vi "SpecFilter.vi"() -> ()   [LabVIEW 2022 SP3]
uses:
  <vilib>/Analysis/NI_AALPro.lvlib
  <vilib>/Analysis/NI_AALBase.lvlib
  <vilib>/Analysis/2dsp.llb/Real FFT.vi
  <vilib>/Analysis/baseanly.llb/Mean (DBL).vi
panel:
  out "Stats":T1 {"Raw ratio" format="%.2f"; "Spec Ratio" format="%.2f"; "Spec SD" format="%.2f"; "Spec mean" format="%.2f"; "Raw SD" format="%.2f"; "Raw mean" format="%.2f"}
  out "Raw Envelope":dbl[][](array[numeric]) format="%.2f"
  out "Spec Data":dbl[][](array[numeric]) format="%.2f"
  out "XY Graph":T2(graph)
  out "Specle Sector image":dbl[][](graph)
  out "Specle Image":dbl[][](graph)
  in  "Log scaling?":bool=TRUE
  in  "Last file opened":path
  out "Sector as data array":dbl[][](graph)
  in  "View Header?":bool
  in  "Header format":u16(ring) items=["Riverside Format", "Ron Linear"]
  out "Raw data":i16[][](graph)
  in  "new file path":path=path "E:/ProstateData/Q162r19.eye"
  # "To view new EYE file delete file path, run application by pushing right pointing arrow, and then choose new file in dialog box."
  # "Ignore if not using a sector scan"
  # "Note columns of the raw data have been inverted\nand the resulting matrix has been transposed to form\nthe sector image. Data reduced from raw form"
  # "© 2000 Riverside Research Institute"
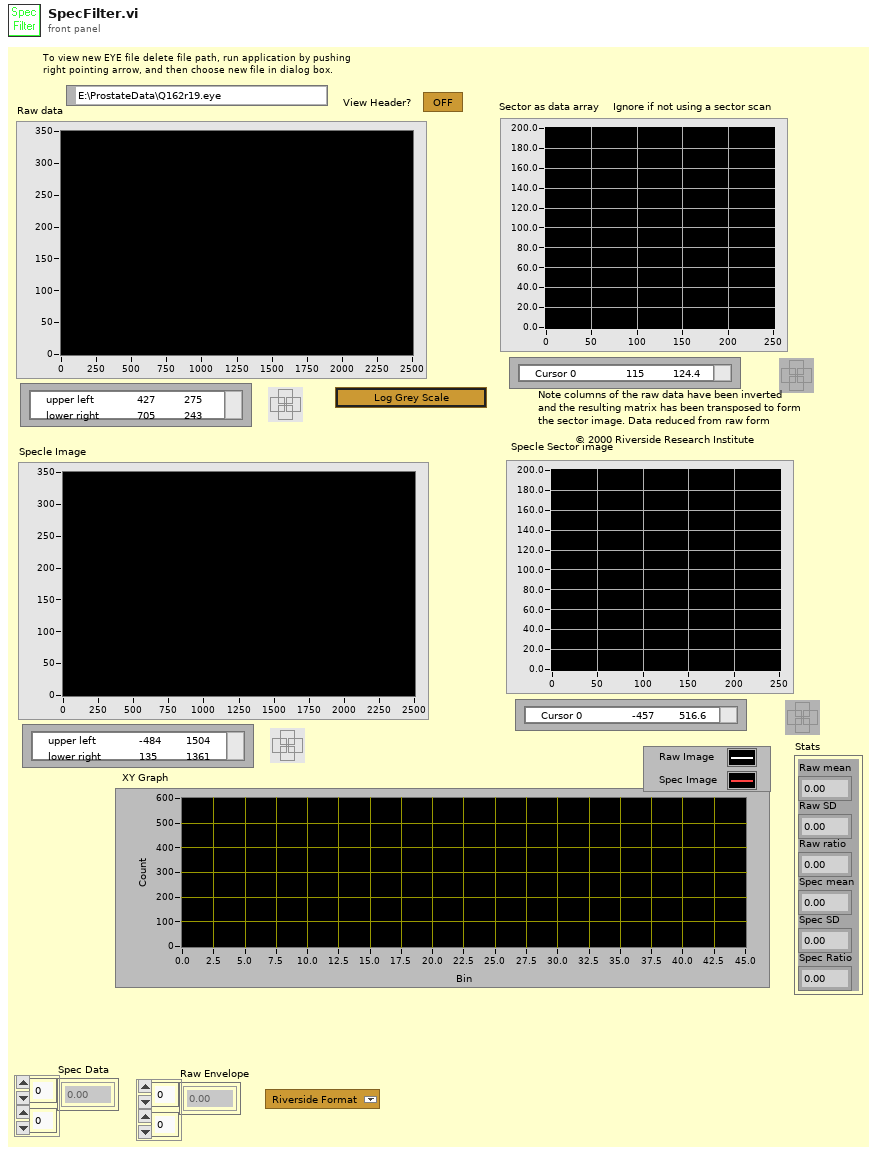
[diagram p1: front panel]
types:
  T1 = cluster{"Raw mean":dbl, "Raw SD":dbl, "Raw ratio":dbl, "Spec mean":dbl, "Spec SD":dbl, "Spec Ratio":dbl}
  T2 = cluster{"X Values":dbl[], "Histogram: h(x)":i32[]}[]
  T3 = cluster{"# rf points per line":u16, "# lines per scan":u16, "sample rate MHz":u16, "# A/D bits":u16, "# bytes per A/D":u16, "TGC Flag":u16, "A/D Type":string}
  T4 = cluster{"bandwidth":sgl, "center freq":sgl, "start freq":sgl, "ID":i32}
  T5 = cluster{"delay":sgl, "pivot distance":sgl, "sector scan angle":sgl, "operator":string, "Scan Mode":string, "location":string}
  T6 = cluster{"X Values":dbl[], "Histogram: h(x)":i32[]}
  T7 = cluster{"mean":dbl, "standard deviation":dbl, dbl, "mean":dbl, "standard deviation":dbl, dbl}
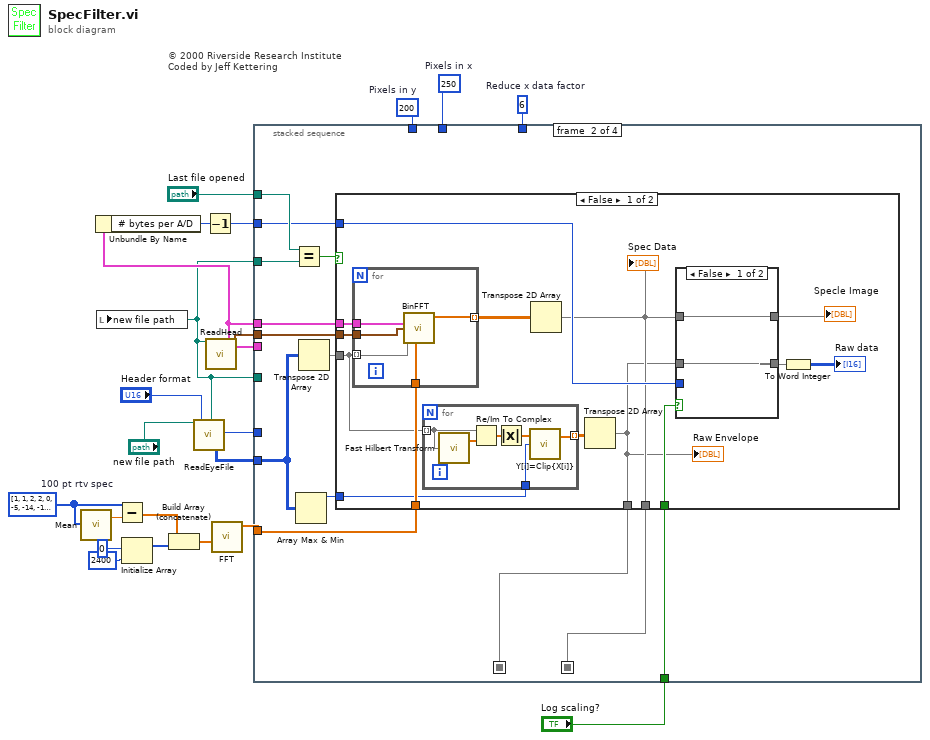
[diagram p0: block diagram]
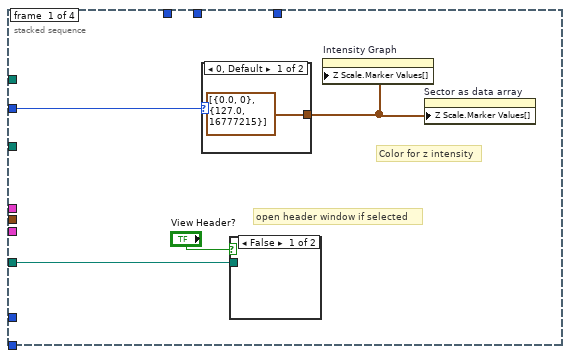
[diagram p2: hidden frame]
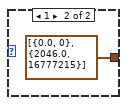
[diagram p3: hidden frame]
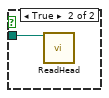
[diagram p4: hidden frame]
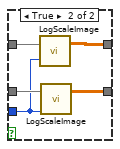
[diagram p5: hidden frame]
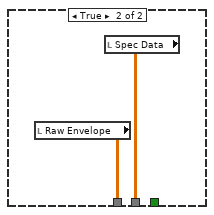
[diagram p6: hidden frame]
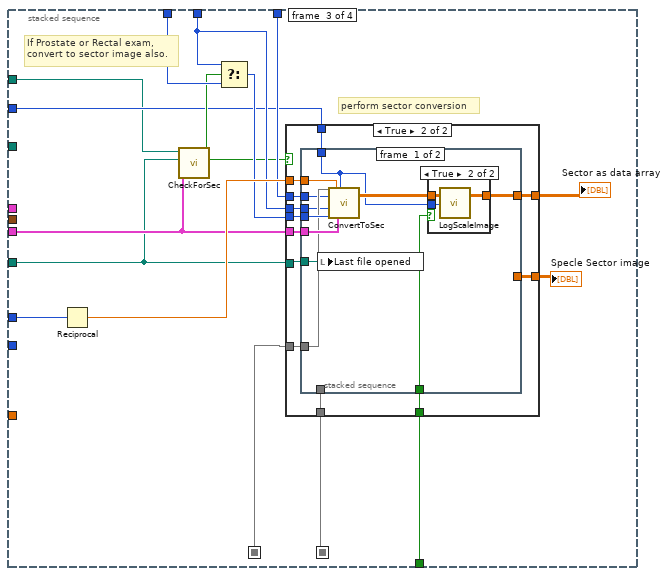
[diagram p7: hidden frame]
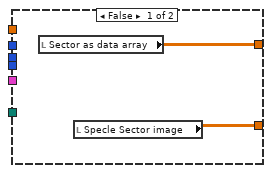
[diagram p8: hidden frame]
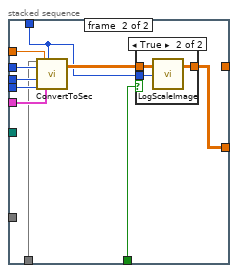
[diagram p10: hidden frame]
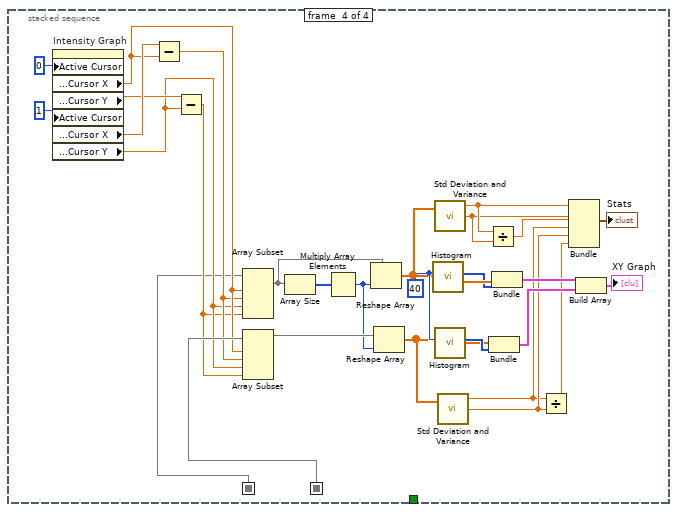
[diagram p12: hidden frame]
diagram:
  w10 = i16[] [1, 1, 2, 2, 0, -5, -14, -15, 1, 31, 52, 42, -4, -58, -81, -58, 2, 62, 88, 70, 20, -31, -56, -51, -27, 3, 20, 22, 14, 6, 0, -3, -5, -6, -7, -6, -3, -2, 0, 2, 3, 2, 1, -1, -3, -4, -3, -2, 1, 2, 2, 2, 1, 0, -1, -1, -1, 0, 1, 1, 1, 1, 1, 1, 1, 0, 0, 0, 0, 0, 1, 1, 1, 1, 1, 0, 0, 0, 0, 1, 1, 1, 1, 1, 1, 1, 1, 0, 0, 1, 1, 1, 1, 1, 1, 0, 0, 0, 0, 0]  # 100 pt rtv spec
  w17 = 6  # Reduce x data factor
  w19 = i16 200  # Pixels in y
  w18 = i16 250  # Pixels in x
  # "© 2000 Riverside Research Institute\nCoded by Jeff Kettering"
  n1 = call-poly <vilib>:"Mean.vi"("X"=w10) -> ("mean"=w12:dbl)  [unwired: 1 out]
  n2 = Subtract(x=w10, y=w12) -> (x-y=w8:dbl[])
  n3 = Initialize Array(0, 2400) -> (w11:i32[])
  n4 = Build Array (concatenate)(w8, w11) -> (w9:dbl[])
  n5 = call "ReadEyeFile.vi"("new file path"="new file path", "Header format"="Header format") -> ("new path out"=w1:path, "2-D data array"=w21:i16[][], "sample rate MHz"=w22:u16)  [unwired: 15 out]
  n6 = local write "new file path"(w1) -> ()
  n7 = call "ReadHead.vi"("new file path"=w1) -> ("A/D info"=w5:T3, "Tranducer Info"=w13:T4, "Scan Info"=w23:T5)  [unwired: 16 out]
  n8 = Unbundle By Name(w5) -> ("# bytes per A/D"=w4:u16)
  n9 = Decrement(x=w4) -> (x-1=w3:u16)
  n10 = call-poly <vilib>:"FFT.vi"("X"=w9) -> ("FFT {X}"=w7:cdb[])  [unwired: 2 in, 8 out]
  n11 = stacked-sequence {
    seq-local: [_ w38 _ _] -> [_ _ w80 w164]
    seq-local: [_ w34 _ _] -> [_ _ w78 w148]
    tunnel: w23 -> [_ _ w88 _]
    tunnel: w22 -> [_ _ w93 _]
    tunnel: w21 -> [_ w32 _ _]
    tunnel: w1 -> [w26 _ w86 _]
    tunnel: w19 -> [_ _ w91 _]
    tunnel: w18 -> [_ _ w90 _]
    tunnel: w17 -> [_ _ w89 _]
    tunnel: w5 -> [_ w43 _ _]
    tunnel: w13 -> [_ w42 _ _]
    tunnel: w7 -> [_ w41 _ _]
    tunnel: "Log scaling?" -> [_ w39 w83 _]
    tunnel: w3 -> [w24 w33 w82 _]
    tunnel: "Last file opened" -> [_ w36 w79 _]
    tunnel: w1 -> [_ w35 _ _]
    frame #0 {
      # "Color for z intensity"
      # "open header window if selected"
      n12 = case shown="0, Default" w24 {
        tunnel: [cluster{dbl, u32}[] [{0.0, 0}, {127.0, 16777215}] ("color scheme 3") cluster{dbl, u32}[] [{0.0, 0}, {2046.0, 16777215}] ("color scheme 3")] -> w25
        frame 0, Default {
        }
        frame 1 {
        }
      }
      n13 = case shown="False" "View Header?" {
        tunnel: w26 -> [_ w30]
        frame False {
        }
        frame True {
          n14 = call "ReadHead.vi"("new file path"=w30) -> ()  [unwired: 19 out]
        }
      }
      n15 = property on="Intensity Graph" class="IntGraph (strict)"("Z Scale.Marker Values[]"=w25) -> ()  [unwired: 2 in, 2 out]
      n16 = property on="Sector as data array" class="IntGraph (strict)"("Z Scale.Marker Values[]"=w25) -> ()  [unwired: 2 in, 2 out]
    }
    frame #1 {
      n17 = Equal?(x=w36, y=w35) -> (x = y?=w37:bool)
      n18 = Array Max & Min(array=w32) -> (max value=w31:i16)  [unwired: 3 out]
      n19 = Transpose 2D Array(2D array=w32) -> (transposed array=w40:i16[][])
      n20 = case shown="False" w37 {
        tunnel: w43 -> [w57 _]
        tunnel: w42 -> [w56 _]
        tunnel: w41 -> [w55 _]
        tunnel: w40 -> [w46 _]
        tunnel: w33 -> [w51 _]
        tunnel: w39 -> [w50 _]
        tunnel: [w48 w77] -> w38
        tunnel: [w47 w76] -> w34
        tunnel: w31 -> [w44 _]
        frame False {
          n21 = for {
            tunnel: w57 -> [w75]
            tunnel: w56 -> [w74]
            tunnel: w55 -> [w73]
            tunnel: w46 -> [w72] mode=indexing
            tunnel: [w71] -> w54 mode=indexing
            n22 = call "BinFFT.vi"("Cal Spectrum"=w73, "RF Data Line"=w72, "Tranducer Info"=w74, "A/D info"=w75) -> ("Envelope of\nOutput bins"=w71:dbl[])  [unwired: 1 in, 6 out]
          }
          n23 = for {
            tunnel: w46 -> [w61] mode=indexing
            tunnel: [w59] -> w45 mode=indexing
            tunnel: w44 -> [w58]
            n24 = call <vilib>:"Fast Hilbert Transform.vi"("X"=w61) -> ("Hilbert{X}"=w62:dbl[])  [unwired: 1 out]
            n25 = Re/Im To Complex(1:w62, 2:w61) -> (0:w63:cdb[])
            n26 = Absolute Value(x=w63) -> (abs(x)=w60:dbl[])
            n27 = call <vilib>:"Y[i]=Clip{X[i]}.vi"("upper limit"=w58, "Input Array"=w60) -> ("Clipped Array"=w59:dbl[])  [unwired: 1 in, 1 out]
          }
          n28 = Transpose 2D Array(2D array=w54) -> (transposed array=w48:dbl[][])
          "Spec Data" <- w48
          n29 = Transpose 2D Array(2D array=w45) -> (transposed array=w47:dbl[][])
          "Raw Envelope" <- w47
          n30 = case shown="False" w50 {
            tunnel: [w64 w70] -> w53
            tunnel: w47 -> [w64 w69]
            tunnel: w51 -> [_ w66]
            tunnel: w48 -> [w65 w68]
            tunnel: [w65 w67] -> w49
            frame False {
            }
            frame True {
              n31 = call "LogScaleImage.vi"("A/D bits"=w66, "input array"=w68) -> ("log scale image"=w67:dbl[][])  [unwired: 1 out]
              n32 = call "LogScaleImage.vi"("A/D bits"=w66, "input array"=w69) -> ("log scale image"=w70:dbl[][])  [unwired: 1 out]
            }
          }
          "Specle Image" <- w49
          n33 = To Word Integer(number=w53) -> (16bit integer=→"Raw data":i16[][])
        }
        frame True {
          n34 = local read "Raw Envelope"() -> (w76:dbl[][])
          n35 = local read "Spec Data"() -> (w77:dbl[][])
        }
      }
    }
    frame #2 {
      # "If Prostate or Rectal exam,\nconvert to sector image also."
      # "perform sector conversion"
      n36 = Reciprocal(x=w93) -> (1/x=w94:dbl)
      n37 = call "CheckForSec.vi"("Scan Info"=w88, "Last sector file opened"=w86, "Current file"=w79) -> ("sector?"=w87:bool, "= 360?"=w84:bool)  [unwired: 5 out]
      n38 = Select(t=w90, s=w84, f=w91) -> (s? t:f=w92:i16)
      n39 = case shown="True" w87 {
        tunnel: [w96 w104] -> w85
        tunnel: w78 -> [_ w102]
        tunnel: w88 -> [_ w108]
        tunnel: w94 -> [_ w107]
        tunnel: w86 -> [_ w106]
        tunnel: w92 -> [_ w105]
        tunnel: w90 -> [_ w99]
        tunnel: w89 -> [_ w100]
        tunnel: w83 -> [_ w103]
        tunnel: w82 -> [_ w101]
        tunnel: [w95 w98] -> w81
        tunnel: w80 -> [_ w97]
        frame False {
          n40 = local read "Sector as data array"() -> (w96:dbl[][])
          n41 = local read "Specle Sector image"() -> (w95:dbl[][])
        }
        frame True {
          n42 = stacked-sequence {
            tunnel: w108 -> [w119 w133]
            tunnel: w107 -> [w118 w132]
            tunnel: w106 -> [w117 _]
            tunnel: w105 -> [w116 w131]
            tunnel: [w115 _] -> w104
            tunnel: w103 -> [w113 w129]
            tunnel: w102 -> [w112 _]
            tunnel: w101 -> [w111 w128]
            tunnel: w100 -> [w110 w127]
            tunnel: w99 -> [w109 w126]
            tunnel: [_ w125] -> w98
            tunnel: w97 -> [_ w124]
            frame #0 {
              n43 = local write "Last file opened"(w117) -> ()
              n44 = call "ConvertToSec.vi"("raw image data in"=w112, "reduce pts by factor of"=w110, "pixels in x"=w109, "pixels in y"=w116, "Time between rf pts\nmicros"=w118, "Scan Info"=w119, "Abs?"=w111) -> ("raw sector out"=w114:dbl[][])  [unwired: 4 in, 8 out]
              n45 = case shown="True" w113 {
                tunnel: [w120 w123] -> w115
                tunnel: w114 -> [w120 w122]
                tunnel: w111 -> [_ w121]
                frame False {
                }
                frame True {
                  n46 = call "LogScaleImage.vi"("A/D bits"=w121, "input array"=w122) -> ("log scale image"=w123:dbl[][])  [unwired: 1 out]
                }
              }
            }
            frame #1 {
              n47 = call "ConvertToSec.vi"("raw image data in"=w124, "reduce pts by factor of"=w127, "pixels in x"=w126, "pixels in y"=w131, "Time between rf pts\nmicros"=w132, "Scan Info"=w133, "Abs?"=w128) -> ("raw sector out"=w130:dbl[][])  [unwired: 4 in, 8 out]
              n48 = case shown="True" w129 {
                tunnel: [w134 w137] -> w125
                tunnel: w130 -> [w134 w136]
                tunnel: w128 -> [_ w135]
                frame False {
                }
                frame True {
                  n49 = call "LogScaleImage.vi"("A/D bits"=w135, "input array"=w136) -> ("log scale image"=w137:dbl[][])  [unwired: 1 out]
                }
              }
            }
          }
        }
      }
      "Sector as data array" <- w85
      "Specle Sector image" <- w81
    }
    frame #3 {
      w156 = 40
      n50 = property on="Intensity Graph" class="IntGraph (strict)"("Active Cursor"=u32 0 ("Write Attribute"), "Active Cursor"=u32 1 ("Write Attribute")) -> ("Cursor.Cursor Position:Cursor X"=w163:dbl, "Cursor.Cursor Position:Cursor Y"=w165:dbl, "Cursor.Cursor Position:Cursor X"=w168:dbl, "Cursor.Cursor Position:Cursor Y"=w161:dbl)  [unwired: 2 in, 2 out]
      n51 = Subtract(x=w168, y=w163) -> (x-y=w162:dbl)
      n52 = Subtract(x=w165, y=w161) -> (x-y=w160:dbl)
      n53 = Array Subset(array=w148, index (row)=w163, length (row)=w162, index (col)=w161, length (col)=w160) -> (w147:dbl[][])
      n54 = Array Subset(array=w164, index (row)=w163, length (row)=w162, index (col)=w161, length (col)=w160) -> (w158:dbl[][])
      n55 = Array Size(array=w147) -> (size(s)=w159:i32[])
      n56 = Multiply Array Elements(1:w159) -> (0:w157:i32)
      n57 = Reshape Array(w147, w157) -> (w146:dbl[])
      n58 = Reshape Array(w158, w157) -> (w145:dbl[])
      n59 = call <vilib>:"Histogram.vi"("intervals"=w156, "X"=w146) -> ("X Values"=w155:dbl[], "Histogram: h(x)"=w154:i32[])  [unwired: 8 out]
      n60 = call <vilib>:"Std Deviation and Variance.vi"("X"=w146) -> ("mean"=w143:dbl, "standard deviation"=w142:dbl)  [unwired: 1 in, 1 out]
      n61 = call <vilib>:"Histogram.vi"("intervals"=w156, "X"=w145) -> ("X Values"=w152:dbl[], "Histogram: h(x)"=w153:i32[])  [unwired: 8 out]
      n62 = call <vilib>:"Std Deviation and Variance.vi"("X"=w145) -> ("mean"=w138:dbl, "standard deviation"=w139:dbl)  [unwired: 1 in, 1 out]
      n63 = Divide(x=w143, y=w142) -> (x/y=w140:dbl)
      n64 = Bundle("X Values"=w152, "Histogram: h(x)"=w153) -> (w150:T6)  [unwired: 1 out]
      n65 = Bundle("X Values"=w155, "Histogram: h(x)"=w154) -> (w151:T6)  [unwired: 1 out]
      n66 = Divide(x=w138, y=w139) -> (x/y=w141:dbl)
      n67 = Bundle("mean"=w143, "standard deviation"=w142, w140, "mean"=w138, "standard deviation"=w139, w141) -> (→"Stats":T7)  [unwired: 1 out]
      n68 = Build Array(w151, w150) -> (→"XY Graph":T2)
    }
  }
